vi "WriteDataUseNotifier.vi"(8 "error in (no error)":errorcluster, 10 "Data":T1, 11 "notifier out":refnum<notifier>) -> (0 "error out":errorcluster, 3 "notifier out":refnum<notifier>)   [LabVIEW 2012, in "DataBank.lvclass"]
uses:
  DataBank.lvclass
  DataBank.lvclass/DataBank.ctl
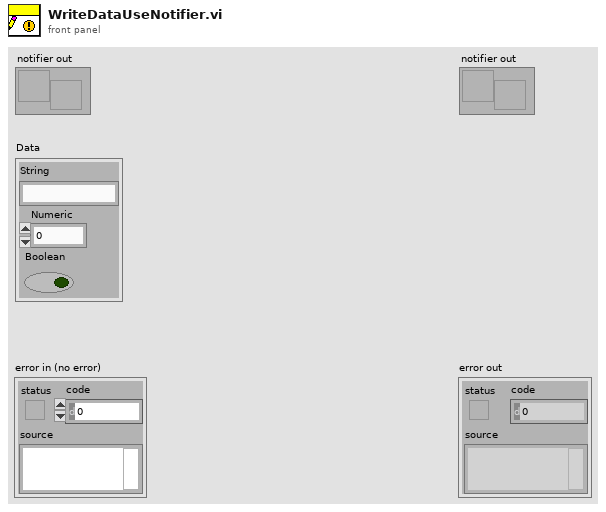
[diagram p1: front panel]
types:
  T1 = cluster{"String":string, "Numeric":i32, "Boolean":bool}
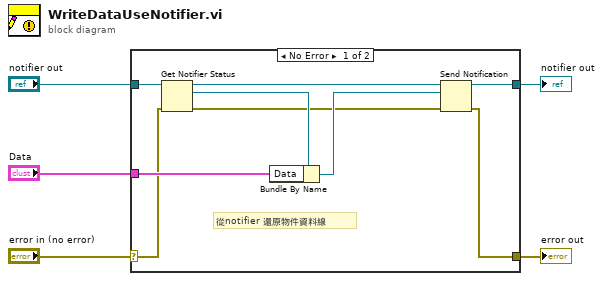
[diagram p0: block diagram]
diagram:
  n1 = case shown="No Error" "error in (no error)" {
    selector: "error in (no error)" -> [w7 w15]
    tunnel: [w6 w15] -> w4
    tunnel: [w10 w16] -> w2
    tunnel: "notifier out" -> [w13 w16]
    tunnel: "Data" -> [w14 _]
    frame No Error {
      # "從notifier 還原物件資料線"
      n2 = Get Notifier Status(notifier=w13, error in (no error)=w7) -> (notifier out=w11:refnum<notifier>, current notification=w12:refnum<class "DataBank.lvclass">, error out=w8:errorcluster)  [unwired: 2 out]
      n3 = Bundle By Name(cluster=w12, "Data"=w14) -> (w9:refnum<class "DataBank.lvclass">)
      n4 = Send Notification(notification=w9, notifier=w11, error in (no error)=w8) -> (notifier out=w10:refnum<notifier>, error out=w6:errorcluster)
    }
    frame Error {
    }
  }
  "error out" <- w4
  "notifier out" <- w2
